vi "Get Server State.vi"(8 "error in":errorcluster, 11 "gRPC server in":refnum<class "Servicer.lvclass">) -> (0 "error out":errorcluster, 2 "Server Internal State":T1, 3 "gRPC server out":refnum<class "Servicer.lvclass">)   [LabVIEW 2019, in "gRPC-servicer.lvlib" / "Servicer.lvclass"]
uses:
  Servicer.lvclass
  typeDefs/Server State Data.ctl
  Servicer.lvclass/Servicer.ctl
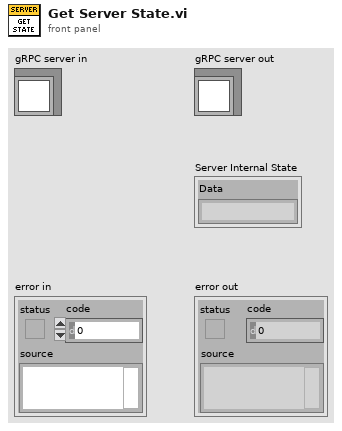
[diagram p1: front panel]
types:
  T1 = typedef "gRPC-servicer.lvlib/Servicer.lvclass/Server State Data.ctl" = cluster{"Data":string}
  T2 = typedef "Template Server.lvlib/Template Server.lvclass/Server State Data.ctl" = cluster{"Data":string}
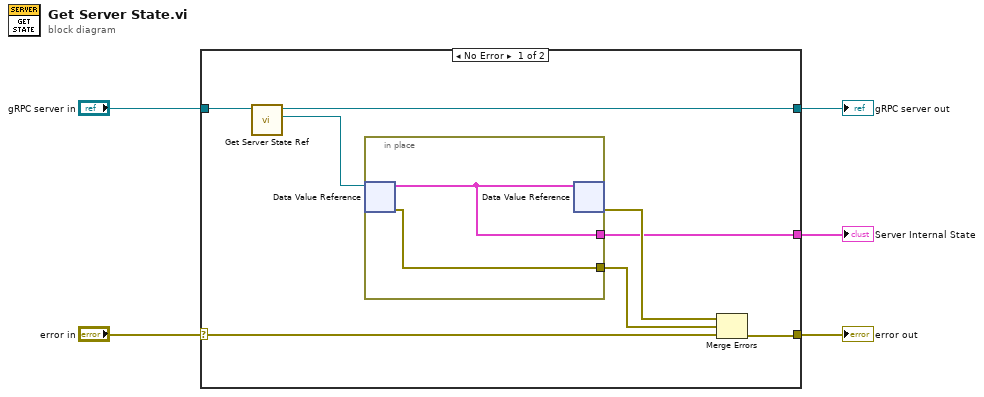
[diagram p0: block diagram]
diagram:
  n1 = case shown="No Error" "error in" {
    selector: "error in" -> [w13 w17]
    tunnel: [w10 w17] -> w4
    tunnel: [w8 w16] -> w2
    tunnel: "gRPC server in" -> [w9 w16]
    tunnel: [w6 _] -> w1
    frame No Error {
      n2 = call "Get Server State Ref.vi"("gRPC server in"=w9) -> ("Server State Ref"=w7:refnum<data-value>, "gRPC server out"=w8:refnum<class "Servicer.lvclass">)  [unwired: 9 in]
      n3 = in-place {
        in-place-border: [w14] -> w6
        in-place-border: [w15] -> w11
        n4 = in-place-dvr #1(w7) -> (w14:T2, w15:errorcluster)
        n5 = in-place-dvr #1(w14) -> (w12:errorcluster)  [unwired: 1 out]
      }
      n6 = Merge Errors(w12, w11, w13) -> (w10:errorcluster)
    }
    frame Error {
    }
  }
  "error out" <- w4
  "gRPC server out" <- w2
  "Server Internal State" <- w1
